vi "SS_Wait4FTP.vi"(6 "Main Cluster IN":T1, 8 "Error In":errorcluster, 11 "Info In":string="\nWaiting for TimerScope Trigger\n- IN: SS TimerScope Trigger\n- OUT: SET SS ThermoRec Received Trigger\nPulse Number is 231123\nPulse Type is 4\n\nDuration (s) is  2.000000\nDelay (s)  is  1.000000\nScan Period (ms) is  15\nNumber of Samples is  134\n\nDelay Started\nDelay Complete\nExternal Measurement of Delay (s): 1.000000\nACQUIRING DATA") -> (0 "Error Out":errorcluster, 3 "Info Out":string="\nWaiting for TimerScope Trigger\n- IN: SS TimerScope Trigger\n- OUT: SET SS ThermoRec Received Trigger\nPulse Number is 231123\nPulse Type is 4\n\nDuration (s) is  2.000000\nDelay (s)  is  1.000000\nScan Period (ms) is  15\nNumber of Samples is  134\n\nDelay Started\nDelay Complete\nExternal Measurement of Delay (s): 1.000000\nACQUIRING DATA", 4 "Main Cluster OUT":T1)   [LabVIEW 2016]
uses:
  Control/Control_Main.ctl
  Control/Control_ModuleArray.ctl
  <vilib>/Platform/TimedLoop/XDataNode/timing_clust.ctl
  <vilib>/Platform/TimedLoop/XDataNode/nitl_modes.ctl
  <vilib>/Platform/TimedLoop/XDataNode/wakeup.ctl
  <vilib>/Platform/TimedLoop/XDataNode/XDataNode.xnode
  <vilib>/Platform/TimedLoop/XDataNode/XDNodeRunTimeDep.lvlib
panel:
  in  "Tab Control":enum32{"IN", "OUT", "SubVI Info"}(tab)
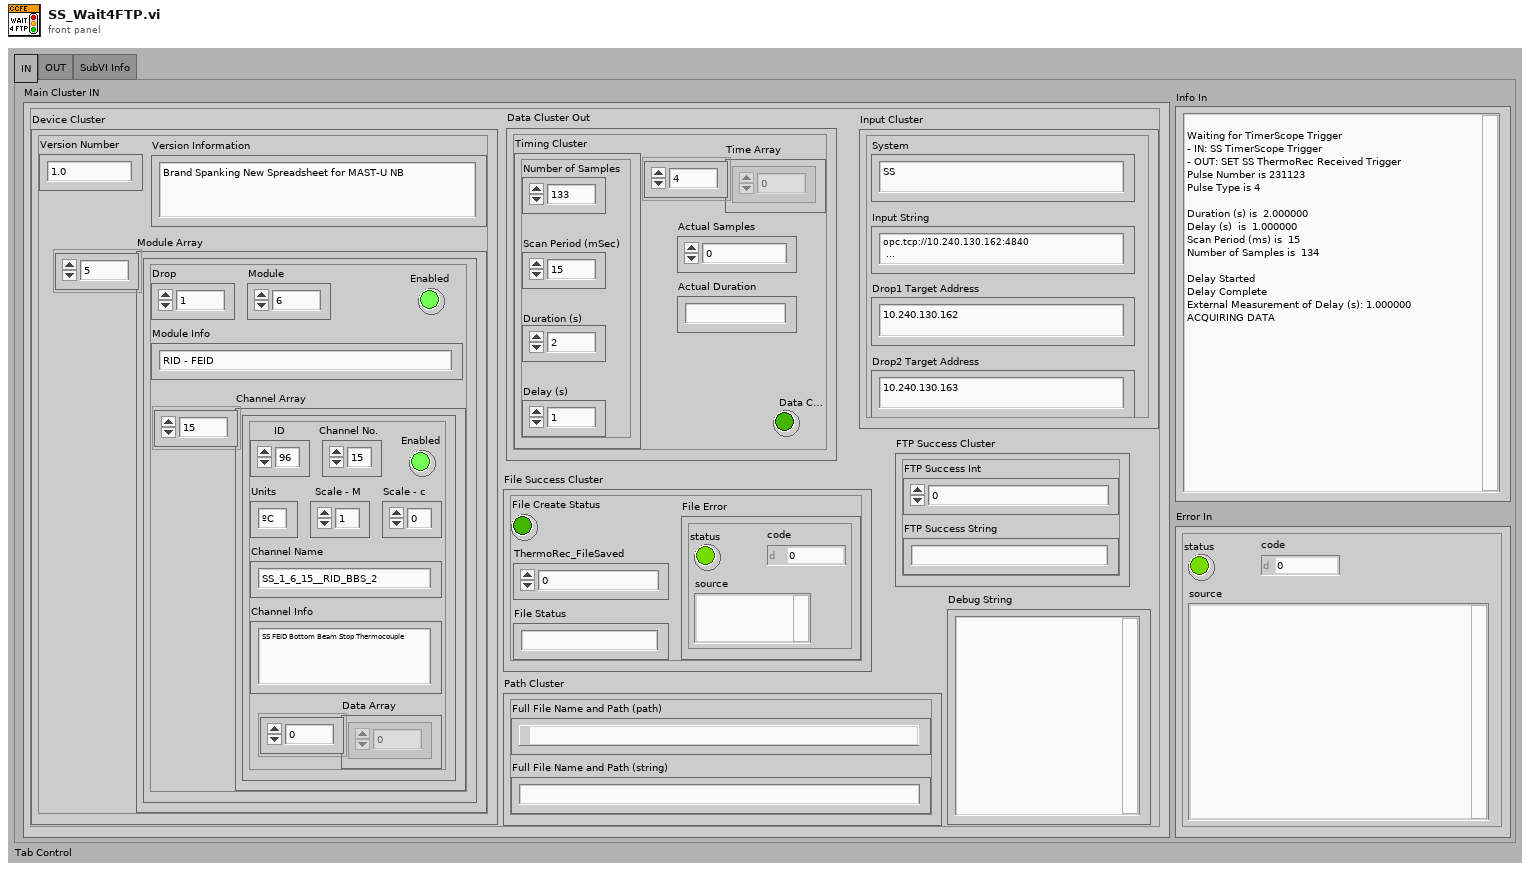
[diagram p1: front panel]
types:
  T1 = typedef "Control_Main.ctl" = cluster{"Device Cluster":cluster{"Module Array":T2, "Version Number":string, "Version Information":string}, "Input Cluster":cluster{"Input String":string, "Drop1 Target Address":string, "Drop2 Target Address":string, "System":string}, "Data Cluster Out":cluster{"Timing Cluster":cluster{"Number of Samples":i32, "Scan Period (mSec)":u32, "Duration (s)":dbl, "Delay (s)":dbl}, "Time Array":dbl[], "Actual Samples":i32, "Actual Duration":string, "Data Collection Error":bool}, "Path Cluster":cluster{"Full File Name and Path (path)":path, "Full File Name and Path (string)":string}, "File Success Cluster":cluster{"ThermoRec_FileSaved":i32, "File Create Status":bool, "File Error":errorcluster, "File Status":string}, "FTP Success Cluster":cluster{"FTP Success Int":i32, "FTP Success String":string}, "Debug String":string}
  T2 = typedef "Control_ModuleArray.ctl" = cluster{"Drop":i32, "Module":i32, "Module Info":string, "Enabled":bool, "Channel Array":cluster{"ID":i32, "Channel No.":i32, "Enabled":bool, "Channel Name":string, "Channel Info":string, "Units":string, "Scale - M":dbl, "Scale - c":dbl, "Data Array":dbl[]}[]}[]
  T3 = typedef "XDNodeRunTimeDep.lvlib/timing_clust.ctl" = cluster{"Expected End [f-1]":u64, "Actual End [f-1]":u64, "Finished Late? [f-1]":bool, "Expected End [i-1]":u64, "Actual End [i-1]":u64, "Finished Late? [i-1]":bool, "Expected Start [i]":u64, "Actual Start [i]":u64, "Expected Start [f]":u64, "Actual Start [f]":u64, "Source Name":string, "Structure Name":string, "Period":i64, "Deadline":i64, "Offset":i64, "Start":i64, "Priority":i32, "Timeout":i32, "Mode":T4, "Wakeup Reason":T5, "Error":errorcluster, "Source Type":string, "Secondary Source Type":string, "Global End Time":u64, "Global Start Time":u64, "Frame Duration":u64, "Iteration Duration":u64, "Assigned CPU":i32, "I/O Scan Engine Mode":u32}
  T4 = typedef "XDNodeRunTimeDep.lvlib/nitl_modes.ctl" = enum32{"No Change", "Process missed periods, maintain original phase", "Discard missed periods, maintain original phase", "Process missed periods, ignore original phase", "Discard missed periods, ignore original phase"}
  T5 = typedef "XDNodeRunTimeDep.lvlib/wakeup.ctl" = enum32{"Normal", "Aborted", "Asynchronous wakeup", "Timing source error", "Timed loop error", "Timeout"}
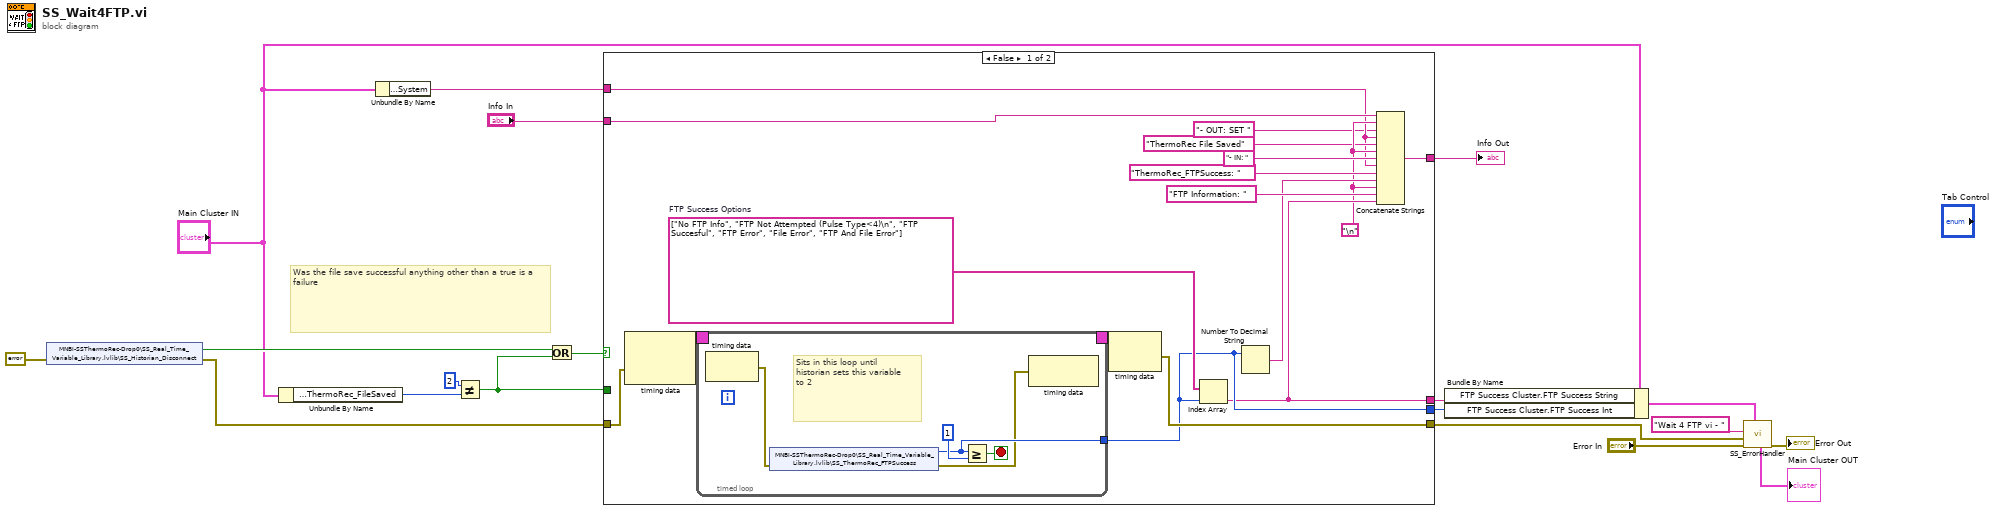
[diagram p0: block diagram]
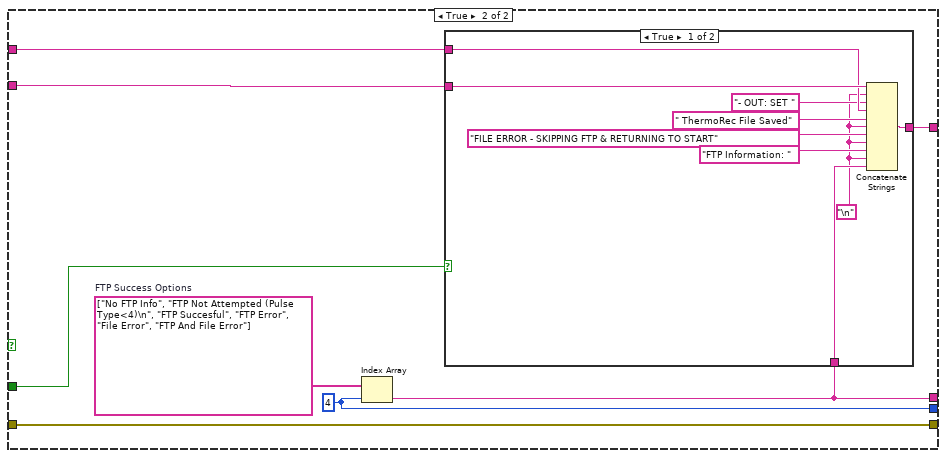
[diagram p2: hidden frame]
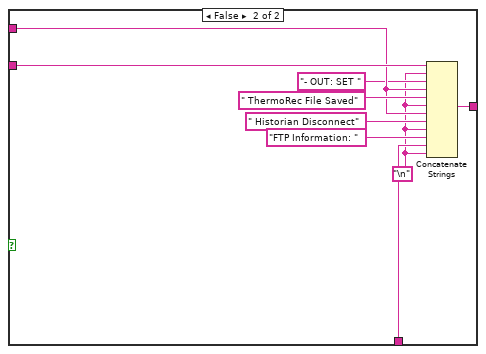
[diagram p3: hidden frame]
diagram:
  # "Was the file save successful anything other than a true is a failure"
  n1 = shared-variable "MNBI-SSThermoRec-Drop0\\SS_Real_Time_Variable_Library.lvlib\\SS_Historian_Disconnect"(error in=errorcluster {"status"=FALSE, "code"=0, "source"=""} ("error constant")) -> (w16:bool, error out=w4:errorcluster)
  n2 = Unbundle By Name("Main Cluster IN") -> ("File Success Cluster.ThermoRec_FileSaved"=w14:i32)
  n3 = Unbundle By Name("Main Cluster IN") -> ("Input Cluster.System"=w2:string)
  n4 = Not Equal?(x=2, y=w14) -> (x != y?=w17:bool)
  n5 = Or(x=w16, y=w17) -> (x .or. y?=w18:bool)
  n6 = case shown="False" w18 {
    tunnel: w4 -> [w31 w58]
    tunnel: [w33 w59] -> w9
    tunnel: [w30 w58] -> w7
    tunnel: "Info In" -> [w32 w57]
    tunnel: w17 -> [_ w53]
    tunnel: [w29 w56] -> w1
    tunnel: [w28 w55] -> w13
    tunnel: w2 -> [w21 w52]
    frame False {
      w36 = string[] ["No FTP Info", "FTP Not Attempted (Pulse Type<4)\n", "FTP Succesful", "FTP Error", "File Error", "FTP And File Error"]  # FTP Success Options
      w23 = "\n"
      n7 = node-c288(w31) -> (w35:T3)  [unwired: 1 in]
      n8 = timed-loop {
        timing: w35 -> [_]
        timing-out: [_] -> w34
        tunnel: [w39] -> w29
        stop <- w41 stop-if-true
        # "Sits in this loop until historian sets this variable to 2"
        n9 = node-c288() -> (w38:errorcluster)  [unwired: 1 in]
        n10 = shared-variable "MNBI-SSThermoRec-Drop0\\SS_Real_Time_Variable_Library.lvlib\\SS_ThermoRec_FTPSuccess"(error in=w38) -> (w39:i32, error out=w37:errorcluster)
        n11 = Greater Or Equal?(x=w39, y=1) -> (x >= y?=w41:bool)
        n12 = node-c288(w37) -> ()  [unwired: 1 out]
      }
      n13 = node-c288(w34) -> (w30:errorcluster)
      n14 = Index Array(array=w36, index=w29) -> (element=w28:string)
      n15 = Number To Decimal String(number=w29) -> (decimal integer string=w26:string)  [unwired: 1 in]
      n16 = Concatenate Strings(w32, w23, "- OUT: SET ", w21, "ThermoRec File Saved", w23, "- IN: ", w21, "ThermoRec_FTPSuccess: ", w26, w23, "FTP Information: ", w28) -> (w33:string)
    }
    frame True {
      w56 = 4
      w54 = string[] ["No FTP Info", "FTP Not Attempted (Pulse Type<4)\n", "FTP Succesful", "FTP Error", "File Error", "FTP And File Error"]  # FTP Success Options
      n17 = Index Array(array=w54, index=w56) -> (element=w55:string)
      n18 = case shown="True" w53 {
        tunnel: [w68 w77] -> w59
        tunnel: w57 -> [w67 w76]
        tunnel: w55 -> [w66 w75]
        tunnel: w52 -> [w62 w71]
        frame True {
          w60 = "\n"
          n19 = Concatenate Strings(w67, w60, "- OUT: SET ", w62, " ThermoRec File Saved", w60, "FILE ERROR - SKIPPING FTP & RETURNING TO START", w60, "FTP Information: ", w60, w66) -> (w68:string)
        }
        frame False {
          w69 = "\n"
          n20 = Concatenate Strings(w76, w69, "- OUT: SET ", w71, " ThermoRec File Saved", w69, w71, " Historian Disconnect", w69, "FTP Information: ", w75, w69) -> (w77:string)
        }
      }
    }
  }
  "Info Out" <- w9
  n21 = Bundle By Name(cluster="Main Cluster IN", "FTP Success Cluster.FTP Success String"=w13, "FTP Success Cluster.FTP Success Int"=w1) -> (w6:T1)
  n22 = call "SS_ErrorHandler.vi"("Main Cluster IN"=w6, "Error In"="Error In", "SubVI Error"=w7, "SubVI Name"="Wait 4 FTP vi - ") -> ("Error Out"=→"Error Out":errorcluster, "Main Cluster OUT"=→"Main Cluster OUT":T1)  [unwired: 5 in, 1 out]
